vi "I2C 6 Axis Gyro Accel LSM6D3.vi"() -> ()   [LabVIEW 2020, in "CTI-Scratchpad.lvlib"]
uses:
  CTI-Scratchpad.lvlib
  CTI/VisaComms/VisaComms.lvclass
  CTI/Session/Session.lvclass
  CTI/GPIO Number.ctl
  CTI/CTI.lvlib
  CTI/I2C Number.ctl
  CTI/Error Reporting.ctl
  CTI-Peripheral/I2C Accel Gyro/Grove 6 Axis Gyro Accel LSM6DS3/Grove 6 Axis Gyro Accel LSM6DS3.lvclass
  CTI/Identity.ctl
panel:
  out "Waveform Chart":T1(graph)
  in  "stop":bool
  out "loop":i32
  out "Identity":T2
  in  "Grove Connector":enum16{"I2C0", "I2C1"}(ring)
  out "error out":errorcluster
  in  "Port":refnum<visa-resource-name>="COM4"
  # "https://wiki.seeedstudio.com/Grove-6-Axis_AccelerometerAndGyroscope/"
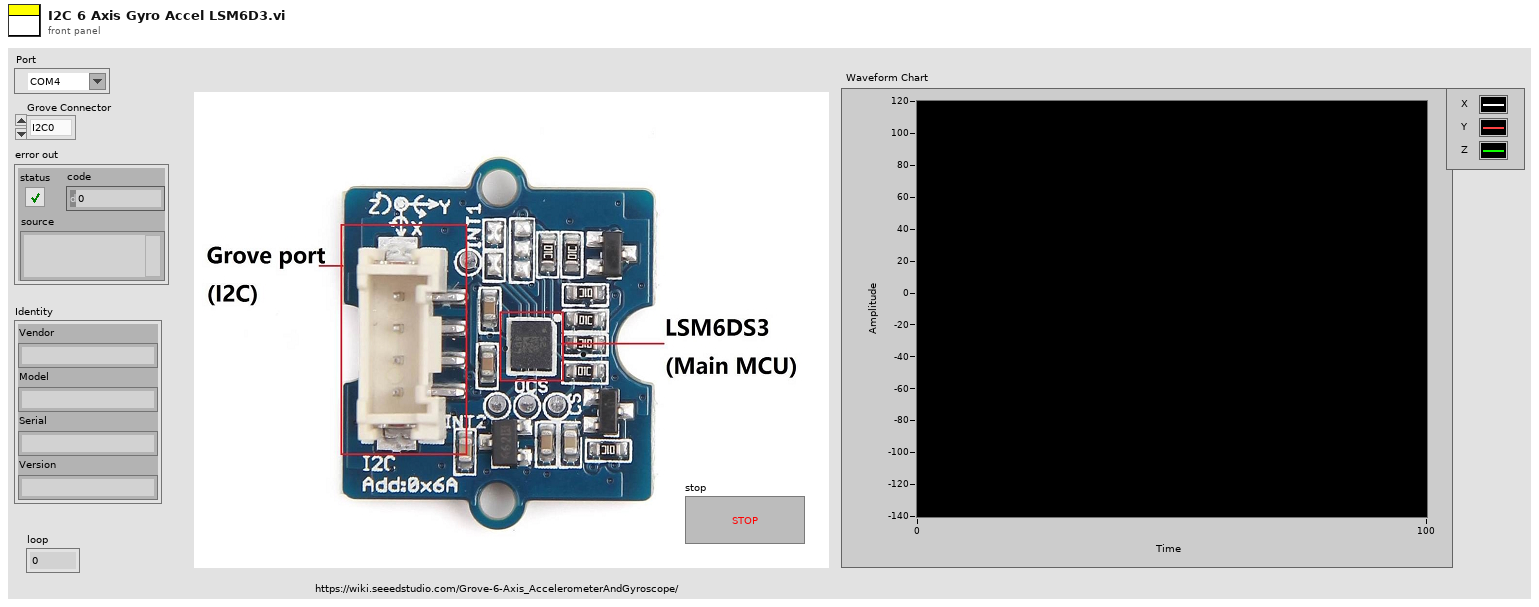
[diagram p1: front panel]
types:
  T1 = cluster{"Array[0]":dbl, "Array[1]":dbl, "Array[2]":dbl}
  T2 = typedef "CTI.lvlib/Identity.ctl" = cluster{"Vendor":string, "Model":string, "Serial":string, "Version":string}
  T3 = typedef "CTI.lvlib/Error Reporting.ctl" = enum16{"Minimal", "Moderate", "Full"}
  T4 = typedef "CTI.lvlib/I2C Number.ctl" = i8
  T5 = typedef "CTI.lvlib/GPIO Number.ctl" = i8
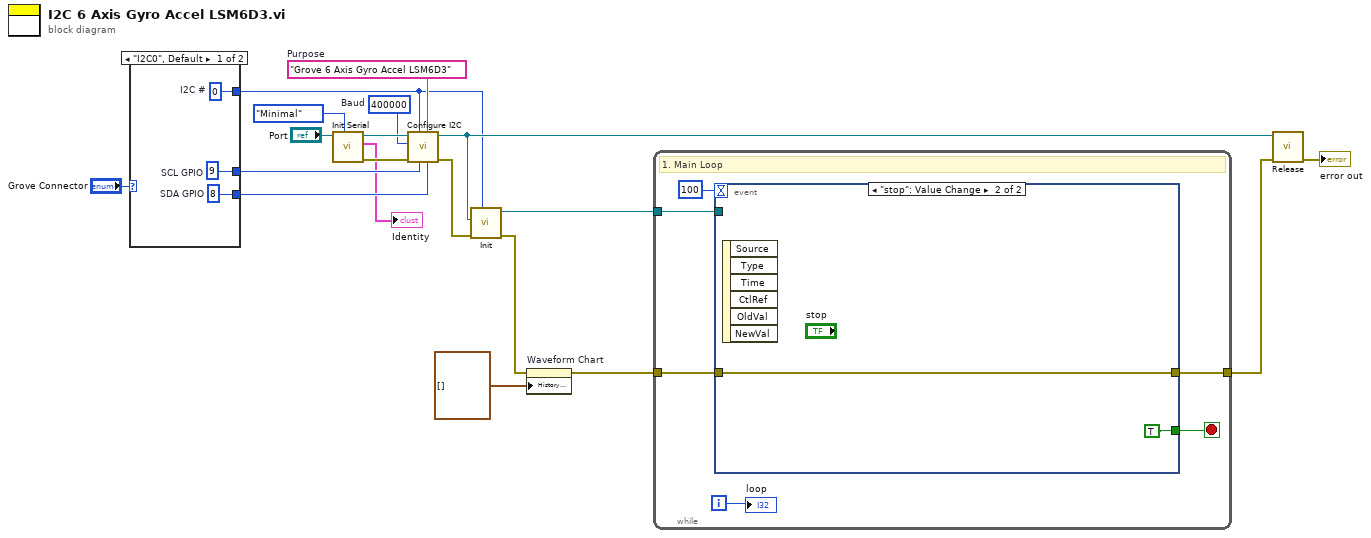
[diagram p0: block diagram]
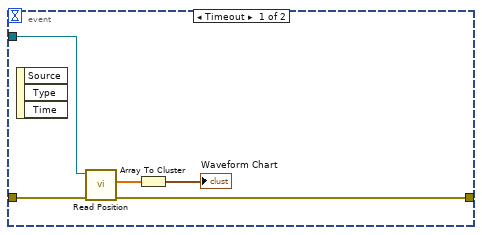
[diagram p2: hidden frame]
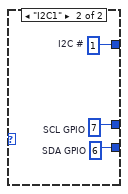
[diagram p3: hidden frame]
diagram:
  w14 = "Grove 6 Axis Gyro Accel LSM6D3"  # Purpose
  w15 = u32 400000  # Baud
  n1 = case shown="\"I2C0\", Default" "Grove Connector" {
    tunnel: [w22 w25] -> w10
    tunnel: [w21 w24] -> w9
    tunnel: [w20 w23] -> w8
    frame "I2C0", Default {
      w20 = T4 0  # I2C #
      w21 = T5 8  # SDA GPIO
      w22 = T5 9  # SCL GPIO
    }
    frame "I2C1" {
      w23 = T4 1  # I2C #
      w24 = T5 6  # SDA GPIO
      w25 = T5 7  # SCL GPIO
    }
  }
  n2 = call "Init Serial.vi"("Error Checking (Full)"=Error_Reporting."Minimal", "VISA resource name in"="Port") -> ("error out"=w16:errorcluster, "Identity"=→"Identity":T2, "Session"=w17:refnum<class "Session.lvclass">)  [unwired: 7 in]
  n3 = call "Configure I2C.vi"("SDA GPIO"=w9, "Purpose (\"I2C\")"=w14, "SCL GPIO"=w10, "I2C #"=w8, "error in (no error)"=w16, "Baud"=w15, "Session in"=w17) -> ("error out"=w13:errorcluster, "Session out"=w12:refnum<class "Session.lvclass">)  [unwired: 3 in]
  n4 = call "Init.vi"("I2C #"=w8, "error in (no error)"=w13, "Session In"=w12) -> ("error out"=w2:errorcluster, "Grove 6 Axis Gyro Accel LSM6DS3 Out"=w6:refnum<class "Grove 6 Axis Gyro Accel LSM6DS3.lvclass">)  [unwired: 7 in]
  n5 = property on="Waveform Chart" class="WFChart (strict)"(error in=w2, "History Data"=cluster{"[0]":dbl, "[1]":dbl, "[2]":dbl}[] []) -> (error out=w1:errorcluster)  [unwired: 1 in, 1 out]
  n6 = while {
    tunnel: w1 -> [w30]
    tunnel: w6 -> [w31]
    tunnel: [w28] -> w5
    i -> [w29]
    stop <- w26 stop-if-true
    # "1. Main Loop"
    n7 = event shown="[1] \"stop\": Value Change" {
      selector: _ -> [_ _]
      dyn-events: _ -> [_ _]
      timeout: 100 -> [_ _]
      tunnel: w31 -> [w35 _]
      tunnel: w30 -> [w36 w37]
      tunnel: [w34 w37] -> w28
      tunnel: [_ TRUE] -> w26
      event Timeout {
        n8 = event-data() -> ()  [unwired: 1 in, 3 out]
        n9 = call-dynamic "Read Position.vi"("error in (no error)"=w36, "Grove 6 Axis Gyro Accel LSM6DS3 in"=w35) -> ("error out"=w34:errorcluster, "Array"=w33:dbl[])  [unwired: 7 in, 1 out]
        n10 = Array To Cluster(array=w33) -> (cluster=→"Waveform Chart":T1)
      }
      event "stop": Value Change {
        n11 = event-data() -> ()  [unwired: 1 in, 6 out]
      }
    }
    "loop" <- w29
  }
  n12 = call-dynamic "Release.vi"("error in (no error)"=w5, "Session in"=w12) -> ("error out"=→"error out":errorcluster)  [unwired: 9 in]
